vi "Read CSV File.vi"(8 "error in (no error)":errorcluster, 11 "Path":path) -> (0 "error out":errorcluster, 2 "Data Out":dbl[](array[numeric]))   [LabVIEW 2022 SP3]
uses:
  <vilib>/Utility/file.llb/Read Delimited Spreadsheet (DBL).vi
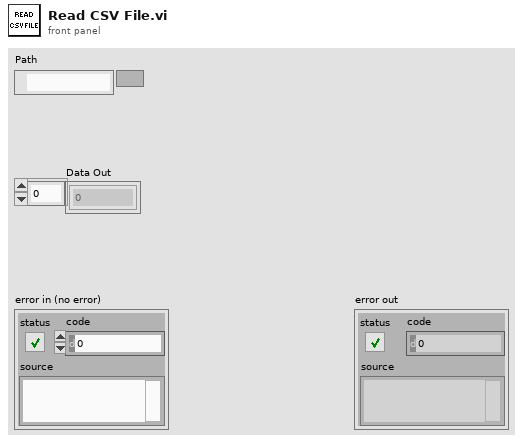
[diagram p1: front panel]
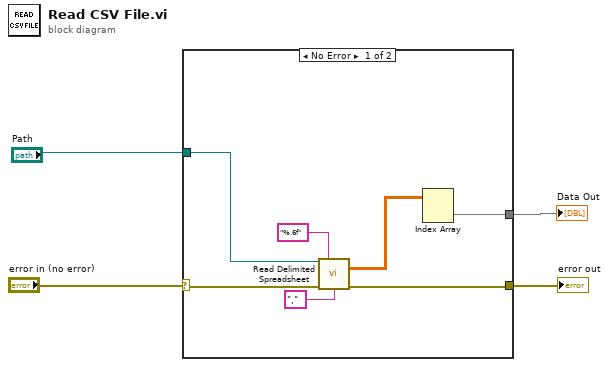
[diagram p0: block diagram]
diagram:
  n1 = case shown="No Error" "error in (no error)" {
    selector: "error in (no error)" -> [w11 w12]
    tunnel: [w10 w12] -> w3
    tunnel: "Path" -> [w9 _]
    tunnel: [w5 _] -> w1
    frame No Error {
      n2 = call-poly <vilib>:"Read Delimited Spreadsheet.vi"("file path (dialog if empty)"=w9, "format (%.3f)"="%.6f", "error in (no error)"=w11, "delimiter (\\t)"="," ("delimiter (\\t)")) -> ("all rows"=w6:dbl[][], "error out"=w10:errorcluster)  [unwired: 6 in, 4 out]
      n3 = Index Array(array=w6) -> (element=w5:dbl[])  [unwired: 2 in]
    }
    frame Error {
    }
  }
  "error out" <- w3
  "Data Out" <- w1
